vi "wrap.PushNumber.vi"(0 "class.GLue in":refnum<class "class.GLue.lvclass">, 7 "Numeric":dbl, 11 "error in (no error)":errorcluster) -> (4 "class.GLue out":refnum<class "class.GLue.lvclass">, 15 "error out":errorcluster)   [LabVIEW 2014, in "GLue.lvlib" / "class.GLue.lvclass"]
uses:
  class.GLue.lvclass
  class.GLue.lvclass/class.GLue.ctl
  Resources/GLue.dll
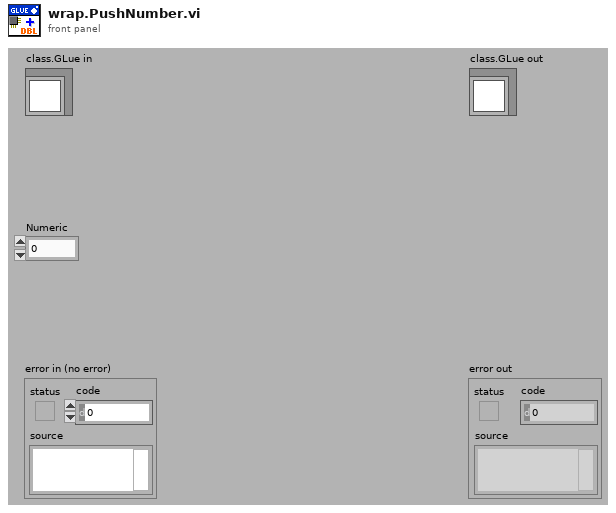
[diagram p1: front panel]
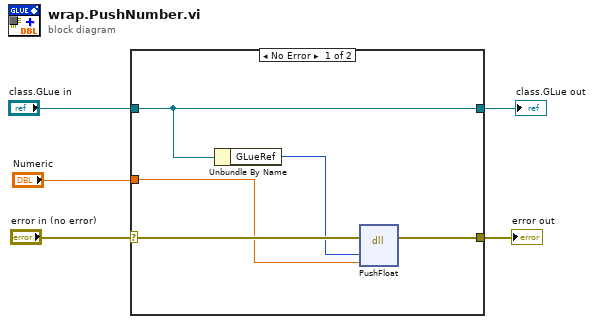
[diagram p0: block diagram]
diagram:
  n1 = case shown="No Error" "error in (no error)" {
    selector: "error in (no error)" -> [w9 w12]
    tunnel: [w8 w12] -> w4
    tunnel: [w10 w11] -> w2
    tunnel: "class.GLue in" -> [w10 w11]
    tunnel: "Numeric" -> [w6 _]
    frame No Error {
      n2 = Unbundle By Name(w10) -> ("GLueRef"=w7:i64)
      n3 = dll-call lib="C:/Users/Antonie/Documents/work/glue/trunk/Resources/GLue.dll" fn="PushFloat"(error in=w9, "GLue"=w7, "double"=w6) -> (error out=w8:errorcluster)  [unwired: 5 in, 1 out]
    }
    frame Error {
    }
  }
  "error out" <- w4
  "class.GLue out" <- w2
